vi "offset.vi"() -> ()   [LabVIEW 2018]
panel:
  in  "cam.tilt.offset.b":dbl=2.4
  in  "cam.tilt.offset.a":dbl=1.0
  in  "cam.pan.offset.b":dbl=1.7
  in  "cam.pan.offset.a":dbl=1.0
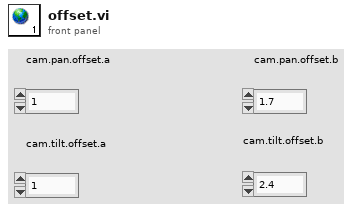
[diagram p1: front panel]
diagram:
